vi "FillScanFuncTree.vi"(6 "AddSymbol(True)":bool=TRUE, 8 "ErrorIn(No Error)":errorcluster caption="entrée d'erreur (pas d'erreur)", 9 "Active ScanPar":bool[](array[boolean]), 10 "ScanFunc":string[][](array[string]), 11 "ScanTreeRef":refnum<vi>) -> (0 "sortie d'erreur":errorcluster, 1 "Active ScanParOut":bool[](array[boolean]))   [LabVIEW 2019]
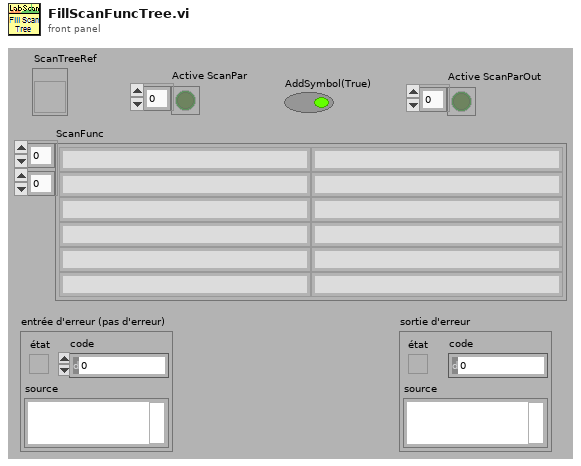
[diagram p1: front panel]
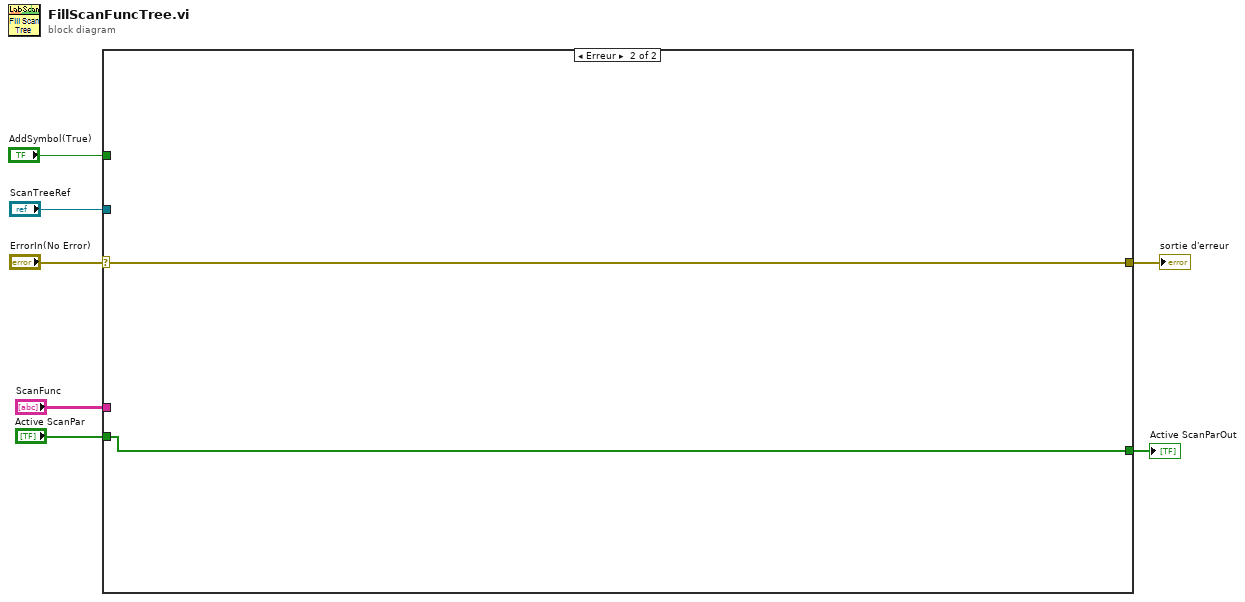
[diagram p0: block diagram]
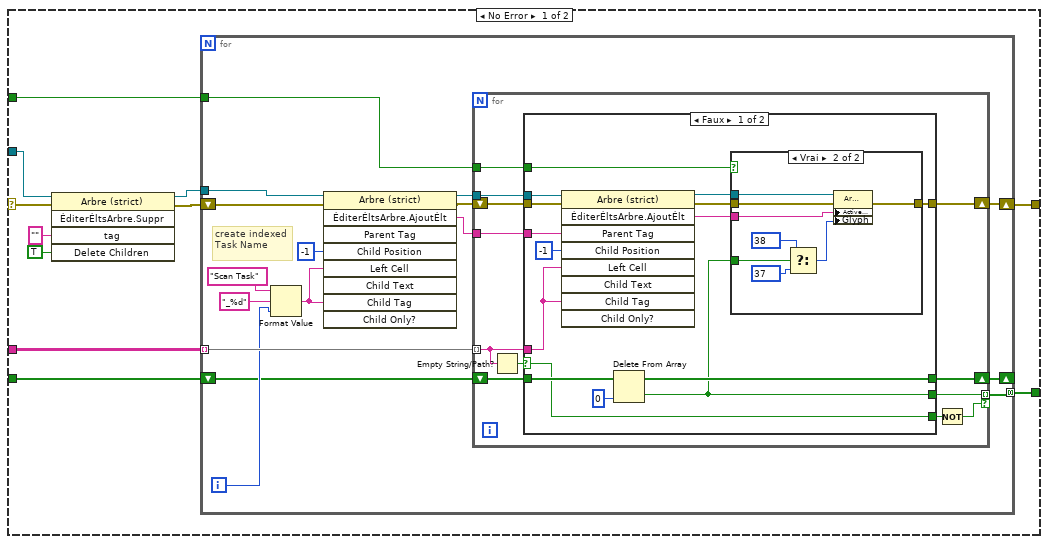
[diagram p2: hidden frame]
diagram:
  n1 = case shown="Erreur" "ErrorIn(No Error)" {
    selector: "ErrorIn(No Error)" -> [w16 w75]
    tunnel: [w17 w75] -> w6
    tunnel: "ScanFunc" -> [w18 _]
    tunnel: "ScanTreeRef" -> [w15 _]
    tunnel: "Active ScanPar" -> [w10 w74]
    tunnel: "AddSymbol(True)" -> [w9 _]
    tunnel: [w8 w74] -> w1
    frame No Error {
      n2 = invoke on="Nœud de méthode" class="Arbre (strict)" method="ÉditerÉltsArbre.Suppr"(reference=w15, error in=w16, "tag"="" ("Tag"), "Delete Children"=TRUE ("Supprimer les enfants ?")) -> (reference out=w14:refnum<vi>, error out=w13:errorcluster)  [unwired: 1 in, 3 out]
      n3 = for {
        tunnel: w18 -> [w34] mode=indexing
        tunnel: w14 -> [w23]
        shift-right: [w25] -> w17
        shift-left: w13 -> [w30]
        shift-right: [w21] -> _
        shift-left: w10 -> [w22]
        tunnel: w9 -> [w20]
        tunnel: [w19] -> w8 mode=concatenating
        i -> [w31]
        # "create indexed Task Name"
        n4 = Format Value(string ("")="Scan Task" ("ClassName"), format string="_%d" ("chaîne de format"), value (0)=w31) -> (output string=w29:string)
        n5 = invoke on="Nœud de méthode" class="Arbre (strict)" method="ÉditerÉltsArbre.AjoutÉlt"(reference=w23, error in=w30, "Child Position"=-1 ("Position de l'enfant"), "Left Cell"=w29, "Child Tag"=w29) -> (reference out=w28:refnum<vi>, error out=w27:errorcluster, "Edit Tree Items:Add Item"=w26:string)  [unwired: 4 in, 6 out]
        n6 = for {
          tunnel: w34 -> [w41] mode=indexing
          tunnel: w28 -> [w46]
          tunnel: w26 -> [w44]
          shift-right: [w43] -> w25
          shift-left: w27 -> [w45]
          shift-right: [w39] -> w21
          shift-left: w22 -> [w40]
          tunnel: w20 -> [w38]
          tunnel: [w37] -> w19 mode=indexing if=w35
          n7 = Empty String/Path?(string/path=w41) -> (empty?=w42:bool)
          n8 = case shown="Faux" w42 {
            selector: w42 -> [w47 w71]
            tunnel: w41 -> [w57 _]
            tunnel: w46 -> [w61 _]
            tunnel: w45 -> [w60 w73]
            tunnel: w44 -> [w59 _]
            tunnel: [w54 w73] -> w43
            tunnel: w40 -> [w52 w72]
            tunnel: [w50 w72] -> w39
            tunnel: w38 -> [w49 _]
            tunnel: [w48 _] -> w37
            tunnel: [w47 w71] -> w36
            frame False {
              n9 = invoke on="Nœud de méthode" class="Arbre (strict)" method="ÉditerÉltsArbre.AjoutÉlt"(reference=w61, error in=w60, "Parent Tag"=w59, "Child Position"=-1 ("Position de l'enfant"), "Left Cell"=w57, "Child Tag"=w57) -> (reference out=w56:refnum<vi>, error out=w55:errorcluster, "Edit Tree Items:Add Item"=w53:string)  [unwired: 3 in, 6 out]
              n10 = Delete From Array(array=w52, index=0 ("indice")) -> (deleted portion=w48:bool, array with subset deleted=w50:bool[])  [unwired: 1 in]
              n11 = case shown="Vrai" w49 {
                tunnel: w56 -> [_ w70]
                tunnel: w55 -> [w62 w69]
                tunnel: [w62 w68] -> w54
                tunnel: w53 -> [_ w67]
                tunnel: w48 -> [_ w64]
                frame False {
                }
                frame True {
                  n12 = Select(t=38 ("symboles"), s=w64, f=37 ("symboles")) -> (s? t:f=w63:i32)
                  n13 = property class="Arbre (strict)"(reference=w70, error in=w69, "Active Item Tag"=w67, "Glyph"=w63) -> (error out=w68:errorcluster)  [unwired: 1 out]
                }
              }
            }
            frame True {
              # "Chaine vide: ne pas ajouter"
            }
          }
          n14 = Not(x=w36) -> (.not. x?=w35:bool)
        }
      }
    }
    frame Error {
    }
  }
  "sortie d'erreur" <- w6
  "Active ScanParOut" <- w1
